vi "Pre Launch Init.vi"(11 "Device in":refnum<class "Device.lvclass">) -> (0 "error out":errorcluster, 3 "Device out":refnum<class "Device.lvclass">)   [LabVIEW 2020, in "Device.lvlib" / "Device.lvclass"]
doc: "(<B>Filename</B>: Actor Framework.lvlib:Actor.lvclass:Pre Launch Init.vi)\n\nDefines behavior that occurs after the Launch Nested Actor method is invoked but before the actor's Actor Core method begins running.\n\nBy default, this method does nothing. A descendant class may override it to define behavior."
uses:
  Device.lvclass
  <vilib>/ActorFramework/Actor/Actor.lvclass
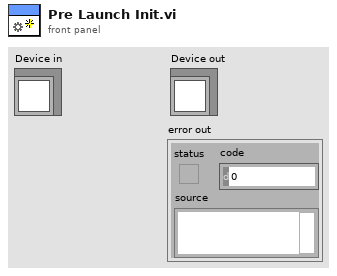
[diagram p1: front panel]
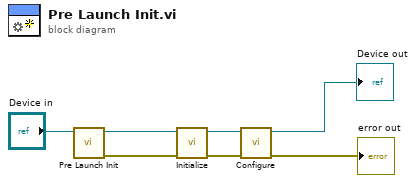
[diagram p0: block diagram]
diagram:
  n1 = call-parent "Pre Launch Init.vi"("Actor in"="Device in") -> ("error out"=w7:errorcluster, "Actor out"=w1:refnum<class "Device.lvclass">)  [unwired: 9 in]
  n2 = call-dynamic "Initialize.vi"("error in (no error)"=w7, "Device in"=w1) -> ("error out"=w5:errorcluster, "Device out"=w3:refnum<class "Device.lvclass">)  [unwired: 8 in]
  n3 = call-dynamic "Configure.vi"("error in (no error)"=w5, "Device in"=w3) -> ("error out"=→"error out":errorcluster, "Device out"=→"Device out":refnum<class "Device.lvclass">)  [unwired: 8 in]
